vi "Get Menu Position.vi"(6 "Position":T1(ring), 7 "VI Refnum(Calling VI)":refnum<vi>, 8 "error in (no error)":errorcluster, 11 "Menu Refnum":refnum<vi>) -> (0 "error out":errorcluster, 3 "Position":cluster{"Top":i16, "Left":i16})   [LabVIEW 2019, in "Menu Launcher Module.lvlib"]
uses:
  Menu Launcher Module.lvlib
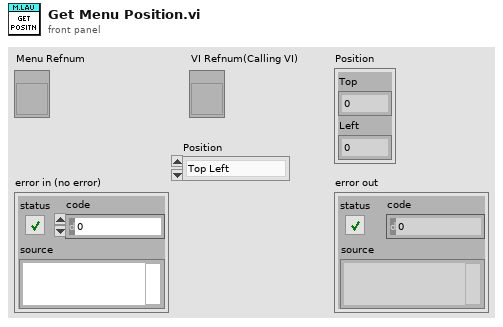
[diagram p1: front panel]
types:
  T1 = enum16{"Top Left", "Top Right", "Bottom Left", "Bottom Right", "Center"}
  T2 = typedef "LVRectTypeDef.ctl" = cluster{"Left":i16, "Top":i16, "Right":i16, "Bottom":i16}
  T3 = typedef "LVPositionTypeDef.ctl" = cluster{"Left":i32, "Top":i32}
  T4 = typedef "LVBoundsTypeDef.ctl" = cluster{"Width":u32, "Height":u32}
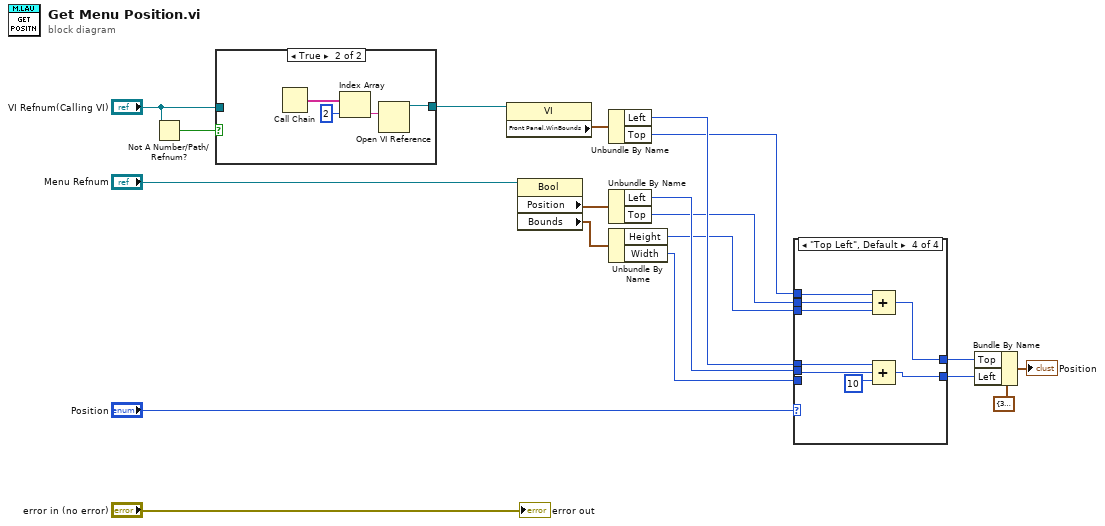
[diagram p0: block diagram]
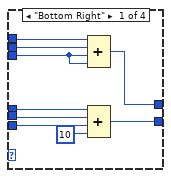
[diagram p2: hidden frame]
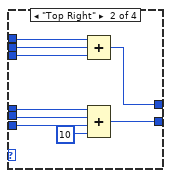
[diagram p3: hidden frame]
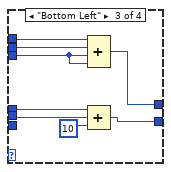
[diagram p4: hidden frame]
diagram:
  n1 = Not A Number/Path/Refnum?(number/path/refnum="VI Refnum(Calling VI)") -> (NaN/Path/Refnum?=w19:bool)
  n2 = case shown="True" w19 {
    tunnel: "VI Refnum(Calling VI)" -> [w20 _]
    tunnel: [w20 w21] -> w16
    frame False {
    }
    frame True {
      n3 = Call Chain() -> (call chain=w24:string[])
      n4 = Index Array(array=w24, index=2) -> (element=w23:string)
      n5 = Open VI Reference(vi path=w23) -> (vi reference=w21:refnum<vi>)  [unwired: 5 in, 1 out]
    }
  }
  n6 = property class="VI"(reference=w16) -> ("Front Panel.WinBounds"=w15:T2)  [unwired: 1 in, 2 out]
  n7 = property on="Property Node" class="Bool"(reference="Menu Refnum") -> ("Position"=w14:T3, "Bounds"=w13:T4)  [unwired: 1 in, 2 out]
  n8 = Unbundle By Name(w15) -> ("Left"=w8:i16, "Top"=w5:i16)
  n9 = Unbundle By Name(w14) -> ("Left"=w7:i32, "Top"=w4:i32)
  n10 = Unbundle By Name(w13) -> ("Height"=w3:u32, "Width"=w6:u32)
  n11 = case shown="\"Top Left\", Default" "Position" {
    tunnel: w8 -> [w33 w42 w50 w58]
    tunnel: w7 -> [w32 w41 w49 w57]
    tunnel: w6 -> [w31 w40 _ _]
    tunnel: w5 -> [w29 w38 w47 w55]
    tunnel: w4 -> [w28 w37 w46 w54]
    tunnel: w3 -> [w27 w36 w45 w53]
    tunnel: [w26 w35 w44 w52] -> w2
    tunnel: [w25 w34 w43 w51] -> w1
    frame "Bottom Right" {
      n12 = Compound Arithmetic op=ADD(w29, w28, w27, w27) -> (w25:u32)
      n13 = Compound Arithmetic op=ADD(w33, w32, w31, u32 10 ("value")) -> (w26:u32)
    }
    frame "Top Right" {
      n14 = Compound Arithmetic op=ADD(w38, w37, w36) -> (w34:u32)
      n15 = Compound Arithmetic op=ADD(w42, w41, w40, u32 10 ("value")) -> (w35:u32)
    }
    frame "Bottom Left" {
      n16 = Compound Arithmetic op=ADD(w47, w46, w45, w45) -> (w43:u32)
      n17 = Compound Arithmetic op=ADD(w50, w49, u32 10 ("value")) -> (w44:u32)
    }
    frame "Top Left", Default {
      n18 = Compound Arithmetic op=ADD(w55, w54, w53) -> (w51:u32)
      n19 = Compound Arithmetic op=ADD(w58, w57, u32 10 ("value")) -> (w52:u32)
    }
  }
  n20 = Bundle By Name(cluster=cluster{"Top":i16, "Left":i16} {"Top"=370, "Left"=710} ("Position"), "Top"=w1, "Left"=w2) -> (→"Position":cluster{"Top":i16, "Left":i16})
  "error out" <- "error in (no error)"
